vi "Periodic Tasks.vi"(8 "error in":errorcluster, 11 "pt cluster":T3={"linear acuator left"={"DeviceStatus"={"status"=FALSE, "code"=0, "source"=""}, "Type"=enum."CAN", "PWM"={"PWM Channel"=enum."Invalid", "DeadBand"={"Name"="", "maxPositivePwm"=0, "minPositivePwm"=0, "centerPwm"=0, "maxNegativePwm"=0, "minNegativePwm"=0, "angularRange"=0}}, "CAN"={"Device Number"=5, "SetOutput VI Ref"=variant(refnum<vi> refnum), "GetOutput VI Ref"=variant(refnum<vi> refnum), "Enable VI Ref"=variant(refnum<vi> refnum), "Disable VI Ref"=variant(refnum<vi> refnum), "Data"=variant(cluster{"Ext ID":u32, "Status 0 Session Handle":u32, "Status 1 Session Handle":u32, "Param Session Handle":u32, "Param Cache ref":refnum<data-value>, "CAN Timeout":u32, "Status 2 Session Handle":u32, "Status 3 Session Handle":u32, "Inverted No WPILib":bool, "Has Configured Limit Sw":bool, "Has Configured Alt Encoder":bool, "Status 4 Session Handle":u32} {"Ext ID"=33882117, "Status 0 Session Handle"=33657, "Status 1 Session Handle"=33658, "Param Session Handle"=33661, "Param Cache ref"=refnum, "CAN Timeout"=10, "Status 2 Session Handle"=33659, "Status 3 Session Handle"=33660, "Inverted No WPILib"=FALSE, "Has Configured Limit Sw"=FALSE, "Has Configured Alt Encoder"=FALSE, "Status 4 Session Handle"=0})}, "Invert"=FALSE, "DIO PWM"={"PWM \"Enable\" Channel"=enum."Invalid", "DIOChannel"=enum."Invalid", "PWM Rate"=0.0}}, "arm extension"={"DeviceStatus"={"status"=FALSE, "code"=0, "source"=""}, "Type"=enum."CAN", "PWM"={"PWM Channel"=enum."Invalid", "DeadBand"={"Name"="", "maxPositivePwm"=0, "minPositivePwm"=0, "centerPwm"=0, "maxNegativePwm"=0, "minNegativePwm"=0, "angularRange"=0}}, "CAN"={"Device Number"=7, "SetOutput VI Ref"=variant(refnum<vi> refnum), "GetOutput VI Ref"=variant(refnum<vi> refnum), "Enable VI Ref"=variant(refnum<vi> refnum), "Disable VI Ref"=variant(refnum<vi> refnum), "Data"=variant(cluster{"Ext ID":u32, "Status 0 Session Handle":u32, "Status 1 Session Handle":u32, "Param Session Handle":u32, "Param Cache ref":refnum<data-value>, "CAN Timeout":u32, "Status 2 Session Handle":u32, "Status 3 Session Handle":u32, "Inverted No WPILib":bool, "Has Configured Limit Sw":bool, "Has Configured Alt Encoder":bool, "Status 4 Session Handle":u32} {"Ext ID"=33882119, "Status 0 Session Handle"=33677, "Status 1 Session Handle"=33678, "Param Session Handle"=33681, "Param Cache ref"=refnum, "CAN Timeout"=10, "Status 2 Session Handle"=33679, "Status 3 Session Handle"=33680, "Inverted No WPILib"=FALSE, "Has Configured Limit Sw"=FALSE, "Has Configured Alt Encoder"=FALSE, "Status 4 Session Handle"=0})}, "Invert"=FALSE, "DIO PWM"={"PWM \"Enable\" Channel"=enum."Invalid", "DIOChannel"=enum."Invalid", "PWM Rate"=0.0}}, "turret"={"DeviceStatus"={"status"=FALSE, "code"=0, "source"=""}, "Type"=enum."CAN", "PWM"={"PWM Channel"=enum."Invalid", "DeadBand"={"Name"="", "maxPositivePwm"=0, "minPositivePwm"=0, "centerPwm"=0, "maxNegativePwm"=0, "minNegativePwm"=0, "angularRange"=0}}, "CAN"={"Device Number"=9, "SetOutput VI Ref"=variant(refnum<vi> refnum), "GetOutput VI Ref"=variant(refnum<vi> refnum), "Enable VI Ref"=variant(refnum<vi> refnum), "Disable VI Ref"=variant(refnum<vi> refnum), "Data"=variant(cluster{"Ext ID":u32, "Status 0 Session Handle":u32, "Status 1 Session Handle":u32, "Param Session Handle":u32, "Param Cache ref":refnum<data-value>, "CAN Timeout":u32, "Status 2 Session Handle":u32, "Status 3 Session Handle":u32, "Inverted No WPILib":bool, "Has Configured Limit Sw":bool, "Has Configured Alt Encoder":bool, "Status 4 Session Handle":u32} {"Ext ID"=33882121, "Status 0 Session Handle"=33651, "Status 1 Session Handle"=33652, "Param Session Handle"=33655, "Param Cache ref"=refnum, "CAN Timeout"=10, "Status 2 Session Handle"=33653, "Status 3 Session Handle"=33654, "Inverted No WPILib"=FALSE, "Has Configured Limit Sw"=FALSE, "Has Configured Alt Encoder"=FALSE, "Status 4 Session Handle"=0})}, "Invert"=FALSE, "DIO PWM"={"PWM \"Enable\" Channel"=enum."Invalid", "DIOChannel"=enum."Invalid", "PWM Rate"=0.0}}, "hood"={"DeviceStatus"={"status"=FALSE, "code"=0, "source"=""}, "Type"=enum."CAN", "PWM"={"PWM Channel"=enum."Invalid", "DeadBand"={"Name"="", "maxPositivePwm"=0, "minPositivePwm"=0, "centerPwm"=0, "maxNegativePwm"=0, "minNegativePwm"=0, "angularRange"=0}}, "CAN"={"Device Number"=14, "SetOutput VI Ref"=variant(refnum<vi> refnum), "GetOutput VI Ref"=variant(refnum<vi> refnum), "Enable VI Ref"=variant(refnum<vi> refnum), "Disable VI Ref"=variant(refnum<vi> refnum), "Data"=variant(cluster{"Ext ID":u32, "Status 0 Session Handle":u32, "Status 1 Session Handle":u32, "Param Session Handle":u32, "Param Cache ref":refnum<data-value>, "CAN Timeout":u32, "Status 2 Session Handle":u32, "Status 3 Session Handle":u32, "Inverted No WPILib":bool, "Has Configured Limit Sw":bool, "Has Configured Alt Encoder":bool, "Status 4 Session Handle":u32} {"Ext ID"=33882126, "Status 0 Session Handle"=33672, "Status 1 Session Handle"=33673, "Param Session Handle"=33676, "Param Cache ref"=refnum, "CAN Timeout"=10, "Status 2 Session Handle"=33674, "Status 3 Session Handle"=33675, "Inverted No WPILib"=FALSE, "Has Configured Limit Sw"=FALSE, "Has Configured Alt Encoder"=FALSE, "Status 4 Session Handle"=0})}, "Invert"=FALSE, "DIO PWM"={"PWM \"Enable\" Channel"=enum."Invalid", "DIOChannel"=enum."Invalid", "PWM Rate"=0.0}}, "climb brake"={"DevStatus"={"status"=FALSE, "code"=0, "source"=""}, "Pneumatics Control Module"=0, "Forward Solenoid Channel"=enum."Solenoid 4", "Reverse Solenoid Channel"=enum."Solenoid 5"}, "buddy climb"={"DevStatus"={"status"=FALSE, "code"=0, "source"=""}, "Pneumatics Control Module"=0, "Forward Solenoid Channel"=enum."Solenoid 6", "Reverse Solenoid Channel"=enum."Solenoid 7"}, "drivetrain shifter"={"DevStatus"={"status"=FALSE, "code"=0, "source"=""}, "Pneumatics Control Module"=0, "Forward Solenoid Channel"=enum."Solenoid 0", "Reverse Solenoid Channel"=enum."Solenoid 1"}, "hood"={"DevStatus"={"status"=FALSE, "code"=0, "source"=""}, "Pneumatics Control Module"=0, "Forward Solenoid Channel"=enum."Solenoid 1", "Reverse Solenoid Channel"=enum."Invalid"}, "climber encoder"={"DevStatus"={"status"=FALSE, "code"=0, "source"=""}, "EncoderIndex"=enum."Enc 2", "CounterIndex"=enum."Invalid", "DistancePerCount"=1.0, "Decoding Type"=enum."4x"}, "shooter encoder"={"DevStatus"={"status"=FALSE, "code"=0, "source"=""}, "EncoderIndex"=enum."Enc 3", "CounterIndex"=enum."Invalid", "DistancePerCount"=1.0, "Decoding Type"=enum."4x"}, "color sensor"={"I2CDevRef"={"DevStatus"={"status"=FALSE, "code"=0, "source"=""}, "Device Address"=82, "Handle"=54, "I2C Bus"=enum."I2C On-Board"}}, "linear acuator left pot"={"DevStatus"={"status"=FALSE, "code"=0, "source"=""}, "Analog Channel"=enum."AI 0", "Invert Output"=FALSE}, "linear acuator right pot "={"DevStatus"={"status"=FALSE, "code"=0, "source"=""}, "Analog Channel"=enum."AI 1", "Invert Output"=FALSE}, "auto balancer pot"={"DevStatus"={"status"=FALSE, "code"=0, "source"=""}, "Analog Channel"=enum."AI 3", "Invert Output"=FALSE}, "shooter"={"DeviceStatus"={"status"=FALSE, "code"=0, "source"=""}, "Type"=enum."CAN", "PWM"={"PWM Channel"=enum."Invalid", "DeadBand"={"Name"="", "maxPositivePwm"=0, "minPositivePwm"=0, "centerPwm"=0, "maxNegativePwm"=0, "minNegativePwm"=0, "angularRange"=0}}, "CAN"={"Device Number"=10, "SetOutput VI Ref"=variant(refnum<vi> refnum), "GetOutput VI Ref"=variant(refnum<vi> refnum), "Enable VI Ref"=variant(refnum<vi> refnum), "Disable VI Ref"=variant(refnum<vi> refnum), "Data"=variant(cluster{"Ext ID":u32, "Status 0 Session Handle":u32, "Status 1 Session Handle":u32, "Param Session Handle":u32, "Param Cache ref":refnum<data-value>, "CAN Timeout":u32, "Status 2 Session Handle":u32, "Status 3 Session Handle":u32, "Inverted No WPILib":bool, "Has Configured Limit Sw":bool, "Has Configured Alt Encoder":bool, "Status 4 Session Handle":u32} {"Ext ID"=33882122, "Status 0 Session Handle"=33689, "Status 1 Session Handle"=33690, "Param Session Handle"=33693, "Param Cache ref"=refnum, "CAN Timeout"=10, "Status 2 Session Handle"=33691, "Status 3 Session Handle"=33692, "Inverted No WPILib"=FALSE, "Has Configured Limit Sw"=FALSE, "Has Configured Alt Encoder"=FALSE, "Status 4 Session Handle"=0})}, "Invert"=FALSE, "DIO PWM"={"PWM \"Enable\" Channel"=enum."Invalid", "DIOChannel"=enum."Invalid", "PWM Rate"=0.0}}, "hopper"={"DeviceStatus"={"status"=FALSE, "code"=0, "source"=""}, "Type"=enum."CAN", "PWM"={"PWM Channel"=enum."PWM 1", "DeadBand"={"Name"="", "maxPositivePwm"=0, "minPositivePwm"=0, "centerPwm"=0, "maxNegativePwm"=0, "minNegativePwm"=0, "angularRange"=0}}, "CAN"={"Device Number"=12, "SetOutput VI Ref"=variant(refnum<vi> refnum), "GetOutput VI Ref"=variant(refnum<vi> refnum), "Enable VI Ref"=variant(refnum<vi> refnum), "Disable VI Ref"=variant(refnum<vi> refnum), "Data"=variant(cluster{"Library":path, "handle":u64, "Control Mode":u16, "UsageFrame":u32, "RefNumName":string, "arbID":u32} {"Library"=path "libCTRE_PhoenixCCI.so", "handle"=2979961472, "Control Mode"=0, "UsageFrame"=0, "RefNumName"="hopper", "arbID"=33816588})}, "Invert"=FALSE, "DIO PWM"={"PWM \"Enable\" Channel"=enum."Invalid", "DIOChannel"=enum."Invalid", "PWM Rate"=0.0}}, "feeder"={"DeviceStatus"={"status"=FALSE, "code"=0, "source"=""}, "Type"=enum."CAN", "PWM"={"PWM Channel"=enum."PWM 1", "DeadBand"={"Name"="", "maxPositivePwm"=0, "minPositivePwm"=0, "centerPwm"=0, "maxNegativePwm"=0, "minNegativePwm"=0, "angularRange"=0}}, "CAN"={"Device Number"=13, "SetOutput VI Ref"=variant(refnum<vi> refnum), "GetOutput VI Ref"=variant(refnum<vi> refnum), "Enable VI Ref"=variant(refnum<vi> refnum), "Disable VI Ref"=variant(refnum<vi> refnum), "Data"=variant(cluster{"Library":path, "handle":u64, "Control Mode":u16, "UsageFrame":u32, "RefNumName":string, "arbID":u32} {"Library"=path "libCTRE_PhoenixCCI.so", "handle"=3034680992, "Control Mode"=0, "UsageFrame"=0, "RefNumName"="feeder", "arbID"=33816589})}, "Invert"=FALSE, "DIO PWM"={"PWM \"Enable\" Channel"=enum."Invalid", "DIOChannel"=enum."Invalid", "PWM Rate"=0.0}}, "intake"={"DeviceStatus"={"status"=FALSE, "code"=0, "source"=""}, "Type"=enum."CAN", "PWM"={"PWM Channel"=enum."PWM 1", "DeadBand"={"Name"="", "maxPositivePwm"=0, "minPositivePwm"=0, "centerPwm"=0, "maxNegativePwm"=0, "minNegativePwm"=0, "angularRange"=0}}, "CAN"={"Device Number"=15, "SetOutput VI Ref"=variant(refnum<vi> refnum), "GetOutput VI Ref"=variant(refnum<vi> refnum), "Enable VI Ref"=variant(refnum<vi> refnum), "Disable VI Ref"=variant(refnum<vi> refnum), "Data"=variant(cluster{"Library":path, "handle":u64, "Control Mode":u16, "UsageFrame":u32, "RefNumName":string, "arbID":u32} {"Library"=path "libCTRE_PhoenixCCI.so", "handle"=42728016, "Control Mode"=0, "UsageFrame"=0, "RefNumName"="intake", "arbID"=33816591})}, "Invert"=FALSE, "DIO PWM"={"PWM \"Enable\" Channel"=enum."Invalid", "DIOChannel"=enum."Invalid", "PWM Rate"=0.0}}, "auto balance"={"DeviceStatus"={"status"=FALSE, "code"=0, "source"=""}, "Type"=enum."PWM", "PWM"={"PWM Channel"=enum."Invalid", "DeadBand"={"Name"="", "maxPositivePwm"=0, "minPositivePwm"=0, "centerPwm"=0, "maxNegativePwm"=0, "minNegativePwm"=0, "angularRange"=0}}, "CAN"={"Device Number"=0, "SetOutput VI Ref"=variant(refnum<vi> refnum), "GetOutput VI Ref"=variant(refnum<vi> refnum), "Enable VI Ref"=variant(refnum<vi> refnum), "Disable VI Ref"=variant(refnum<vi> refnum), "Data"=variant}, "Invert"=FALSE, "DIO PWM"={"PWM \"Enable\" Channel"=enum."Invalid", "DIOChannel"=enum."Invalid", "PWM Rate"=0.0}}, "linear acuator right"={"DeviceStatus"={"status"=FALSE, "code"=0, "source"=""}, "Type"=enum."CAN", "PWM"={"PWM Channel"=enum."Invalid", "DeadBand"={"Name"="", "maxPositivePwm"=0, "minPositivePwm"=0, "centerPwm"=0, "maxNegativePwm"=0, "minNegativePwm"=0, "angularRange"=0}}, "CAN"={"Device Number"=6, "SetOutput VI Ref"=variant(refnum<vi> refnum), "GetOutput VI Ref"=variant(refnum<vi> refnum), "Enable VI Ref"=variant(refnum<vi> refnum), "Disable VI Ref"=variant(refnum<vi> refnum), "Data"=variant(cluster{"Ext ID":u32, "Status 0 Session Handle":u32, "Status 1 Session Handle":u32, "Param Session Handle":u32, "Param Cache ref":refnum<data-value>, "CAN Timeout":u32, "Status 2 Session Handle":u32, "Status 3 Session Handle":u32, "Inverted No WPILib":bool, "Has Configured Limit Sw":bool, "Has Configured Alt Encoder":bool, "Status 4 Session Handle":u32} {"Ext ID"=33882118, "Status 0 Session Handle"=33662, "Status 1 Session Handle"=33663, "Param Session Handle"=33666, "Param Cache ref"=refnum, "CAN Timeout"=10, "Status 2 Session Handle"=33664, "Status 3 Session Handle"=33665, "Inverted No WPILib"=FALSE, "Has Configured Limit Sw"=FALSE, "Has Configured Alt Encoder"=FALSE, "Status 4 Session Handle"=0})}, "Invert"=FALSE, "DIO PWM"={"PWM \"Enable\" Channel"=enum."Invalid", "DIOChannel"=enum."Invalid", "PWM Rate"=0.0}}} {"color sensor"."I2CDevRef"."Device Address" format="%.0x"}) -> ()   [LabVIEW 2019]
doc: "This VI runs in parallel to other tasks. It can contain as many user-defined periodic loops as you need. These can carry out PID or other sorts of timed response."
uses:
  ptclustergood.ctl
  <vilib>/Rock Robotics/WPI/MotorControl/WPI_MotorControlDeviceRef.ctl
  <vilib>/Rock Robotics/WPI/MotorControl/WPI_MotorControlType.ctl
  <vilib>/Rock Robotics/SystemInterfaces/DIO/FPGA_DIOPWMChannel.ctl
  <vilib>/Rock Robotics/WPI/PWM/WPI_PWMDeadband.ctl
  <vilib>/Rock Robotics/SystemInterfaces/DIO/FPGA_DIOChannel.ctl
  <vilib>/Rock Robotics/WPI/Solenoid/WPI_SolenoidDevRef.ctl
  <vilib>/Rock Robotics/WPI/Solenoid/WPI_SolenoidChannel.ctl
  <vilib>/Rock Robotics/WPI/Encoder/WPI_EncoderDevRef.ctl
  <vilib>/Rock Robotics/SystemInterfaces/Encoder/FPGA_EncoderIdx.ctl
  <vilib>/Rock Robotics/SystemInterfaces/Counter/FPGA_CounterCtrSystemIndex.ctl
  <vilib>/Rock Robotics/WPI/Encoder/WPI_EncoderType.ctl
  <vilib>/Rock Robotics/WPI/ThirdParty/REV Robotics/Color SensorV3/Typedef/Color Sensor V3 DevRef.ctl
  <vilib>/Rock Robotics/WPI/I2C/WPI_I2CDevRef.ctl
  <vilib>/Rock Robotics/SystemInterfaces/i2clib/i2c_bus.ctl
  <vilib>/Rock Robotics/WPI/Potentiometer/WPI_PotentiometerDevRef.ctl
  <vilib>/Rock Robotics/SystemInterfaces/AI/FPGA_AIChannel.ctl
  <vilib>/Rock Robotics/WPI/ThirdParty/REV Robotics/SPARK MAX/Typedef/Spark MAX Control Type.ctl
  GlobalVariables.vi
  <vilib>/Rock Robotics/Network Tables/NT Read Number.vi
  <vilib>/addons/control/pid/pid.llb/PID (DBL).vi
  <vilib>/Rock Robotics/Network Tables/NT Write Number.vi
  <vilib>/addons/control/pid/NI_PID_pid.lvlib
panel:
  out "Shooter in range?":bool
  out "Crash Avoidance":bool
  in  "PID Constants hood":T1={"P Gain"=0.0, "I Gain"=0.0, "D Gain"=0.0, "F Gain"=0.0, "I Zone"=0.0, "Min Output"=-1.0, "Max Output"=1.0} {"Max Output" min=-1.0 max=1.0 step=0.01; "Min Output" min=-1.0 max=1.0 step=0.01; "I Zone" step=0.01; "F Gain" step=0.01; "D Gain" step=0.01; "I Gain" step=0.01; "P Gain" min=0.0 step=0.01}
  in  "offset zone 1":dbl
  in  "offset zone 3":dbl
  in  "setpoint":dbl=4800.0 format="%#_13g"
  in  "shooting":dbl=3.0
  in  "control panel lin act offset":dbl=0.25
  in  "min RPM":dbl=4100.0
  out "Sensor Velocity":dbl
  in  "No Color":cluster{"R":dbl, "G":dbl, "B":dbl}={"R"=80.0, "G"=119.0, "B"=55.0}
  in  "Yellow":cluster{"R":dbl, "G":dbl, "B":dbl}={"R"=83.0, "G"=130.0, "B"=41.0}
  in  "Blue":cluster{"R":dbl, "G":dbl, "B":dbl}={"R"=51.0, "G"=115.0, "B"=88.0}
  in  "Red":cluster{"R":dbl, "G":dbl, "B":dbl}={"R"=103.0, "G"=104.0, "B"=49.0}
  in  "Green":cluster{"R":dbl, "G":dbl, "B":dbl}={"R"=59.0, "G"=132.0, "B"=64.0}
  out "Confidence":dbl=0.9468771343442995
  out "Matched Color Name":string="Red"
  out "Proximity":u16=88
  out "Measured Color":cluster{"R":dbl, "G":dbl, "B":dbl}={"R"=91.53846153846153, "G"=108.97435897435896, "B"=54.48717948717948}
  out "Color":u32(colorbox)=6057270
  in  "PID Constants shooter":T1={"P Gain"=0.00141, "I Gain"=0.0, "D Gain"=0.0, "F Gain"=0.0004, "I Zone"=0.0, "Min Output"=0.0, "Max Output"=1.0} {"Max Output" min=-1.0 max=1.0 step=0.01; "Min Output" min=-1.0 max=1.0 step=0.01; "I Zone" step=0.01; "F Gain" step=0.01; "D Gain" step=0.01; "I Gain" step=0.01; "P Gain" min=0.0 step=0.01}
  in  "protect":dbl=0.2
  in  "offset zone 2":dbl
  in  "trench":dbl=41.3
  in  "layup":dbl=1.0
  in  "Hood Gains":T2={"proportional gain (Kc)"=0.1, "integral time (Ti, min)"=0.0, "derivative time (Td, min)"=0.0} {"derivative time (Td, min)" format="%.3f"; "integral time (Ti, min)" format="%.3f"; "proportional gain (Kc)" format="%.5f"}
  in  "degrees per click hood":dbl=0.278416
  out "hood degrees":dbl=28.823331198364258
  in  "Shooter Gains":T2={"proportional gain (Kc)"=2.0, "integral time (Ti, min)"=0.0, "derivative time (Td, min)"=0.0} {"derivative time (Td, min)" format="%.3f"; "integral time (Ti, min)" format="%.3f"; "proportional gain (Kc)" format="%.3f"}
  in  "lower limit":dbl=-270.0 format="%#_13g"
  in  "upper limit":dbl format="%#_13g"
  in  "Minimum Track Value Turret":dbl=0.05 format="%#_13g"
  in  "Auto Correct Gain Turret":dbl=1.2 format="%#_13g"
  in  "X Accepted Range Turret":dbl
  in  "Backward":dbl
  in  "Forward":dbl=-180.0
  in  "Arm Extension Gains":T2={"proportional gain (Kc)"=0.15, "integral time (Ti, min)"=0.0, "derivative time (Td, min)"=0.0} {"derivative time (Td, min)" format="%.3f"; "integral time (Ti, min)" format="%.3f"; "proportional gain (Kc)" format="%.5f"}
  in  "Turret Gains":T2={"proportional gain (Kc)"=0.025, "integral time (Ti, min)"=0.0, "derivative time (Td, min)"=0.0} {"derivative time (Td, min)" format="%.3f"; "integral time (Ti, min)" format="%.3f"; "proportional gain (Kc)" format="%.5f"}
  in  "degrees per click turret":dbl=1.65
  out "RPM":dbl
  in  "Acuator Gains":T2={"proportional gain (Kc)"=0.3, "integral time (Ti, min)"=0.0, "derivative time (Td, min)"=0.0} {"derivative time (Td, min)" format="%.3f"; "integral time (Ti, min)" format="%.3f"; "proportional gain (Kc)" format="%.5f"}
  in  "right act value at 1 inch":dbl=0.919
  out "right act pos":dbl=-0.2551903082312883
  out "left act pos":dbl=-0.2307307128952676
  in  "left act value at 1 inch":dbl=0.919
  in  "Inches per volt":dbl=13.5
  out "acuator left":dbl=0.936091163918168
  out "acuator right":dbl=0.9379029857949104
  out "turret degrees":dbl=-0.43214263468980785
  in  "clicks per inch arm":dbl=0.251624
  in  "control panel":dbl=5.0
  in  "climb":dbl=10.5
  in  "Ground":dbl=-0.3
  out "Arm Extension Encoder":dbl=5.206198121124268
  in  "climb":dbl=19.0
  in  "control panel":dbl=8.0
  in  "intake":dbl=8.5
  in  "protect":dbl=2.0
  # "Arm Height"
  # "Arm Extension"
  # "Linear Acuator Controls"
  # "Practice Bot\nLeft : .88\nRight : .886\n\nComb Bot\nLeft : .919\nRight : .919"
  # "Shooter"
  # "Click here to set max"
  # "Click here to set min"
  # "Click here to set max"
  # "Click here to set min"
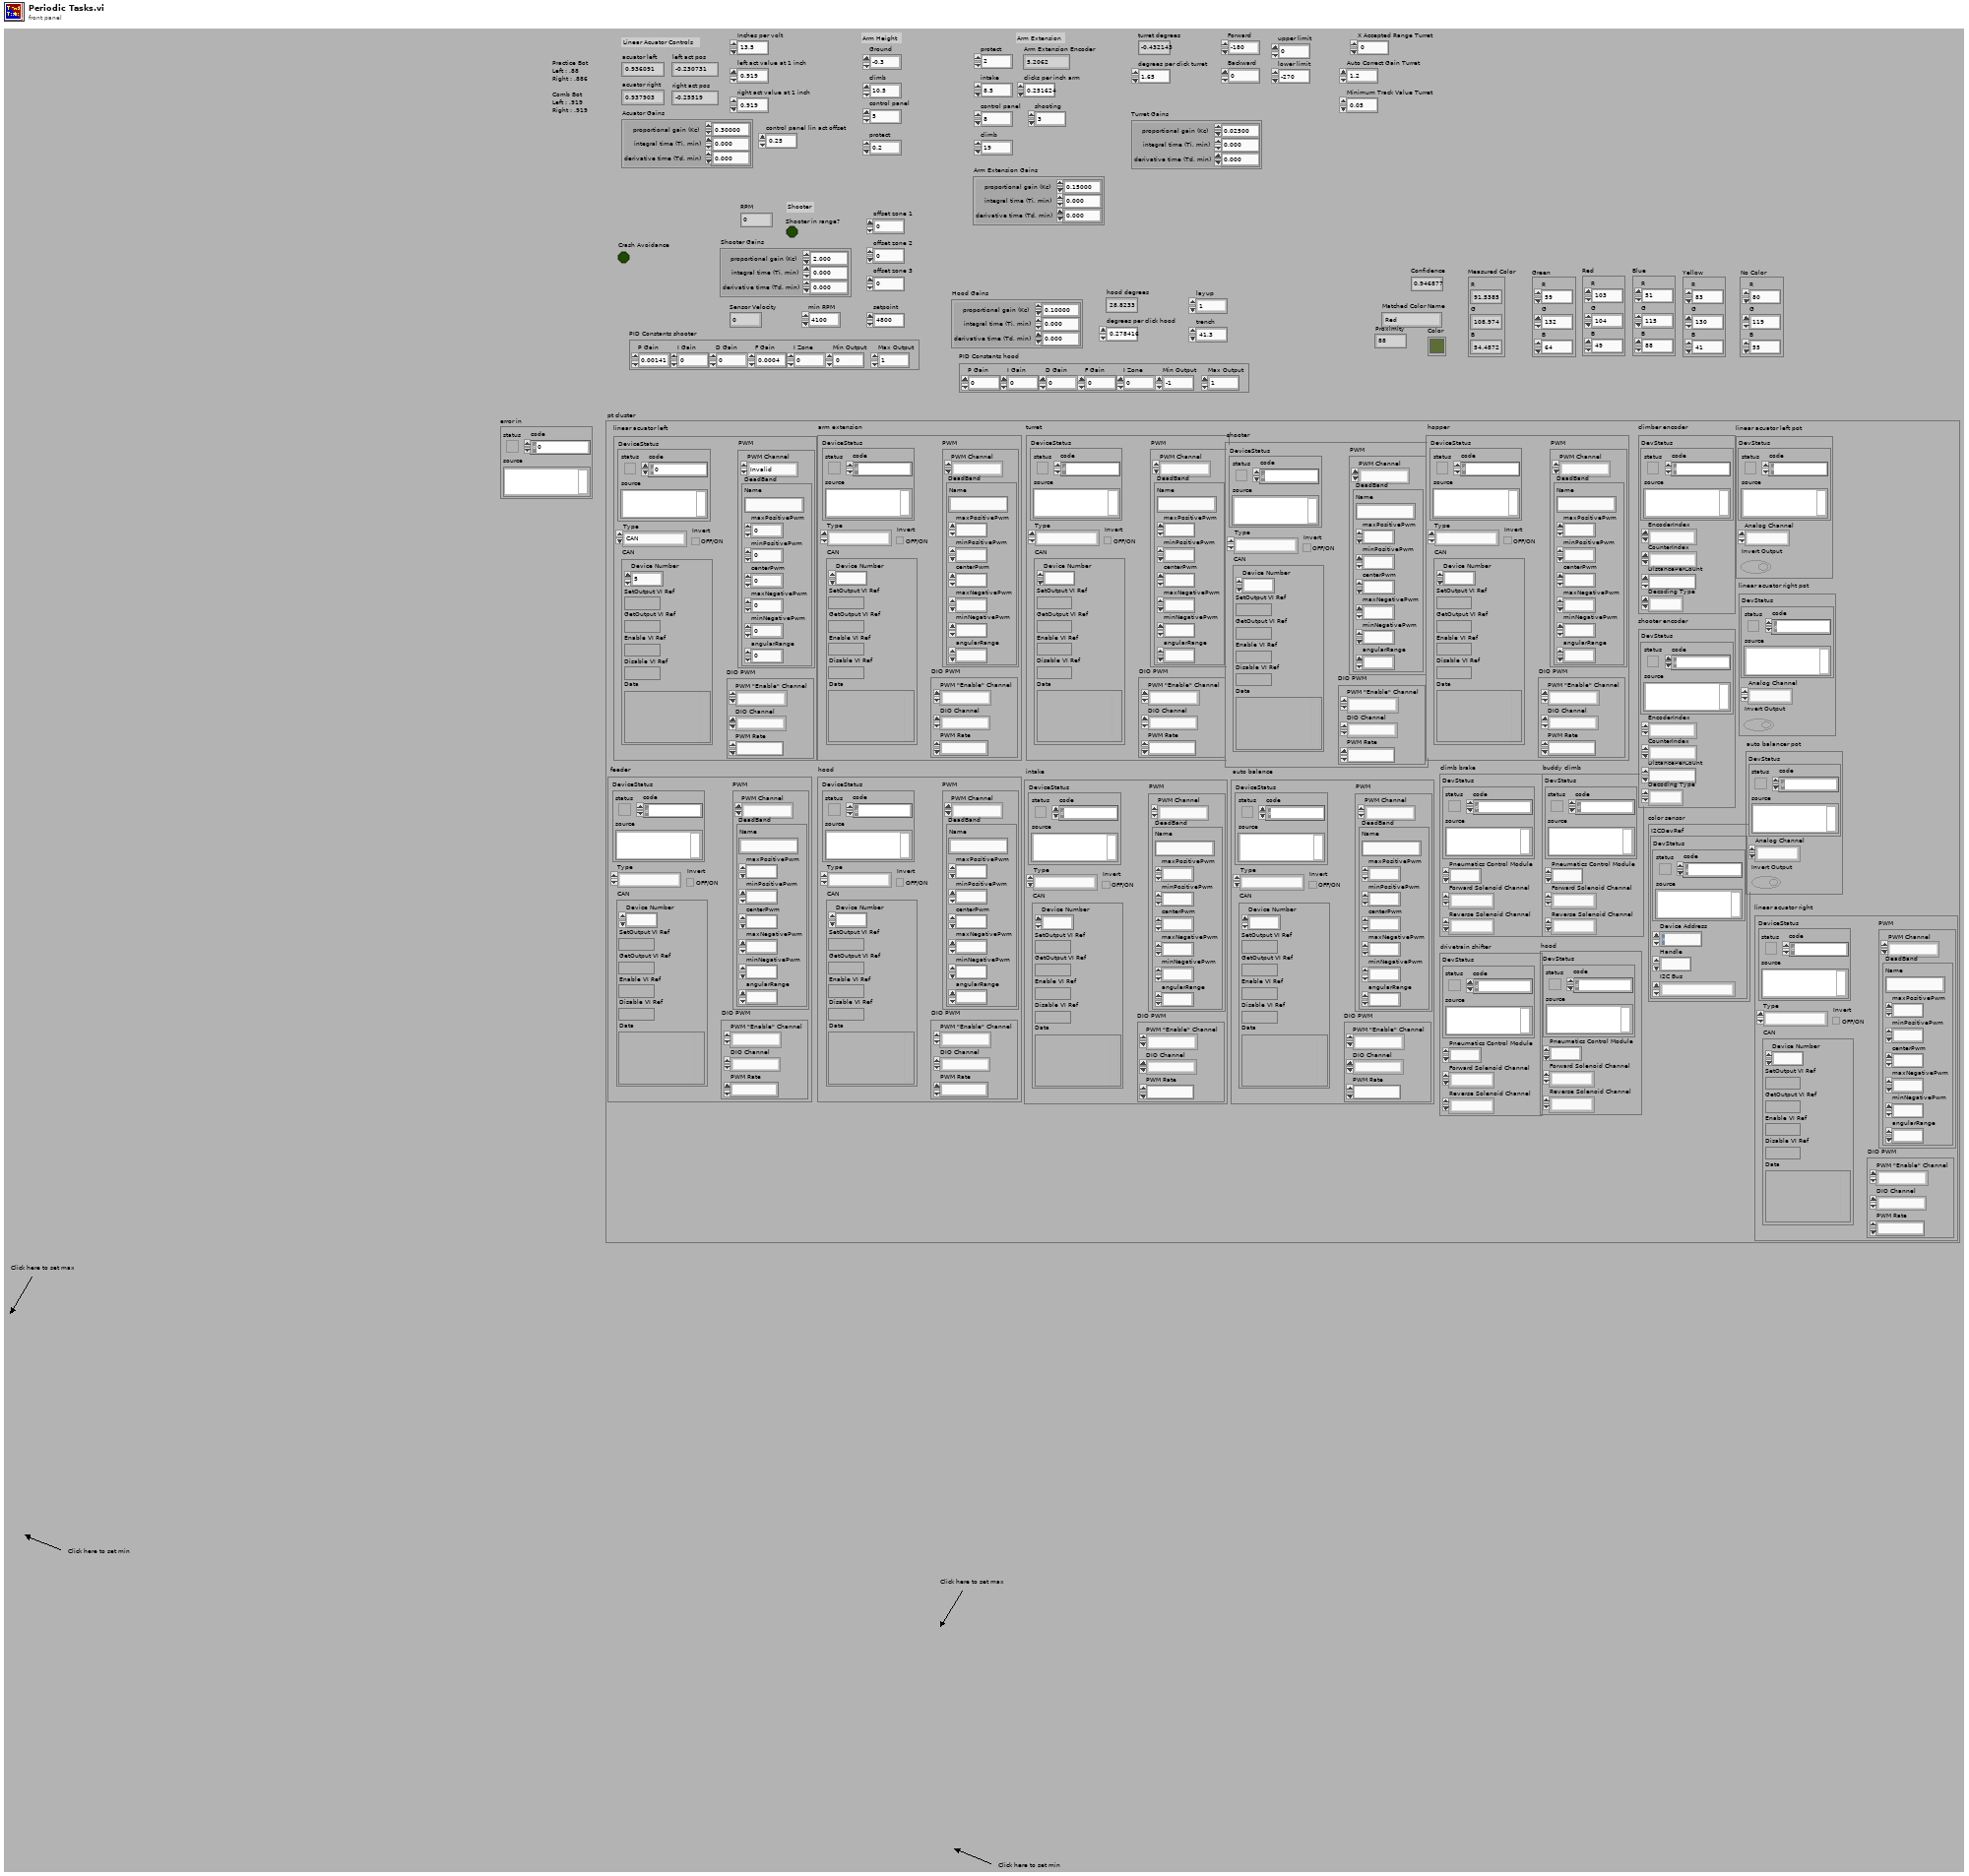
[diagram p1: front panel]
types:
  T1 = cluster{"P Gain":dbl, "I Gain":dbl, "D Gain":dbl, "F Gain":dbl, "I Zone":dbl, "Min Output":dbl, "Max Output":dbl}
  T2 = cluster{"proportional gain (Kc)":dbl, "integral time (Ti, min)":dbl, "derivative time (Td, min)":dbl}
  T3 = typedef "ptclustergood.ctl" = cluster{"linear acuator left":T4, "arm extension":T4, "turret":T4, "hood":T4, "climb brake":T9, "buddy climb":T9, "drivetrain shifter":T9, "hood":T9, "climber encoder":T11, "shooter encoder":T11, "color sensor":T15, "linear acuator left pot":T18, "linear acuator right pot ":T18, "auto balancer pot":T18, "shooter":T4, "hopper":T4, "feeder":T4, "intake":T4, "auto balance":T4, "linear acuator right":T4}
  T4 = typedef "WPI_MotorControlDeviceRef.ctl" = cluster{"DeviceStatus":errorcluster, "Type":T5, "PWM":cluster{"PWM Channel":T6, "DeadBand":T7}, "CAN":cluster{"Device Number":u8, "SetOutput VI Ref":variant, "GetOutput VI Ref":variant, "Enable VI Ref":variant, "Disable VI Ref":variant, "Data":variant}, "Invert":bool, "DIO PWM":cluster{"PWM \"Enable\" Channel":T6, "DIOChannel":T8, "PWM Rate":dbl}}
  T5 = typedef "WPI_MotorControlType.ctl" = enum16{"PWM", "CAN", "DIO PWM"}
  T6 = typedef "FPGA_DIOPWMChannel.ctl" = enum8{"PWM 0", "PWM 1", "PWM 2", "PWM 3", "PWM 4", "PWM 5", "PWM 6", "PWM 7", "PWM 8", "PWM 9", "PWM MXP 0", "PWM MXP 1", "PWM MXP 2", "PWM MXP 3", "PWM MXP 4", "PWM MXP 5", "PWM MXP 6", "PWM MXP 7", "PWM MXP 8", "PWM MXP 9", "Invalid"}
  T7 = typedef "WPI_PWMDeadband.ctl" = cluster{"Name":string, "maxPositivePwm":i32, "minPositivePwm":i32, "centerPwm":i32, "maxNegativePwm":i32, "minNegativePwm":i32, "angularRange":u16}
  T8 = typedef "FPGA_DIOChannel.ctl" = enum8{"DIO 0", "DIO 1", "DIO 2", "DIO 3", "DIO 4", "DIO 5", "DIO 6", "DIO 7", "DIO 8", "DIO 9", "DIO MXP 0", "DIO MXP 1", "DIO MXP 2", "DIO MXP 3", "DIO MXP 4", "DIO MXP 5", "DIO MXP 6", "DIO MXP 7", "DIO MXP 8", "DIO MXP 9", "DIO MXP 10", "DIO MXP 11", "DIO MXP 12", "DIO MXP 13", "DIO MXP 14", "DIO MXP 15", "SPI Port CS1", "SPI Port CS2", "SPI Port CS3", "SPI Port MISO", "SPI Port MOSI", "Invalid"}
  T9 = typedef "WPI_SolenoidDevRef.ctl" = cluster{"DevStatus":errorcluster, "Pneumatics Control Module":u8, "Forward Solenoid Channel":T10, "Reverse Solenoid Channel":T10}
  T10 = typedef "WPI_SolenoidChannel.ctl" = enum8{"Solenoid 0", "Solenoid 1", "Solenoid 2", "Solenoid 3", "Solenoid 4", "Solenoid 5", "Solenoid 6", "Solenoid 7", "Invalid"}
  T11 = typedef "WPI_EncoderDevRef.ctl" = cluster{"DevStatus":errorcluster, "EncoderIndex":T12, "CounterIndex":T13, "DistancePerCount":dbl, "Decoding Type":T14}
  T12 = typedef "FPGA_EncoderIdx.ctl" = enum8{"Enc 0", "Enc 1", "Enc 2", "Enc 3", "Enc 4", "Enc 5", "Enc 6", "Enc 7", "Invalid"}
  T13 = typedef "FPGA_CounterCtrSystemIndex.ctl" = enum8{"Ctr 0", "Ctr 1", "Ctr 2", "Ctr 3", "Ctr 4", "Ctr 5", "Ctr 6", "Ctr 7", "Invalid"}
  T14 = typedef "WPI_EncoderType.ctl" = enum16{"1x", "2x", "4x"}
  T15 = typedef "Color Sensor V3 DevRef.ctl" = cluster{"I2CDevRef":T16}
  T16 = typedef "WPI_I2CDevRef.ctl" = cluster{"DevStatus":errorcluster, "Device Address":u8, "Handle":i32, "I2C Bus":T17}
  T17 = typedef "i2c_bus.ctl" = enum16{"I2C On-Board", "I2C MXP", "Invalid"}
  T18 = typedef "WPI_PotentiometerDevRef.ctl" = cluster{"DevStatus":errorcluster, "Analog Channel":T19, "Invert Output":bool}
  T19 = typedef "FPGA_AIChannel.ctl" = enum8{"AI 0", "AI 1", "AI 2", "AI 3", "AI MXP 0", "AI MXP 1", "AI MXP 2", "AI MXP 3", "Invalid"}
  T20 = typedef "WPI_AnalogChannelDevRef.ctl" = cluster{"DevStatus":errorcluster, "Analog Channel":T19}
  T21 = typedef "Spark MAX Control Type.ctl" = enum16{"Percent VBus", "Voltage", "Velocity", "Position", "Smart Motion", "Current", "Smart Velocity"}
  T22 = enum16{"ground protect", "ground pickup", "control panel", "shooting", "climb", "unjam", "intake shoot"}
  T23 = enum16{"intake", "protect", "control", "climb", "shooting"}
  T24 = enum16{"ground", "protect", "climb", "control panel"}
  T25 = cluster{"P Gain":bool, "I Gain":bool, "D Gain":bool, "F Gain":bool, "I Zone":bool, "Min Output":bool, "Max Output":bool}
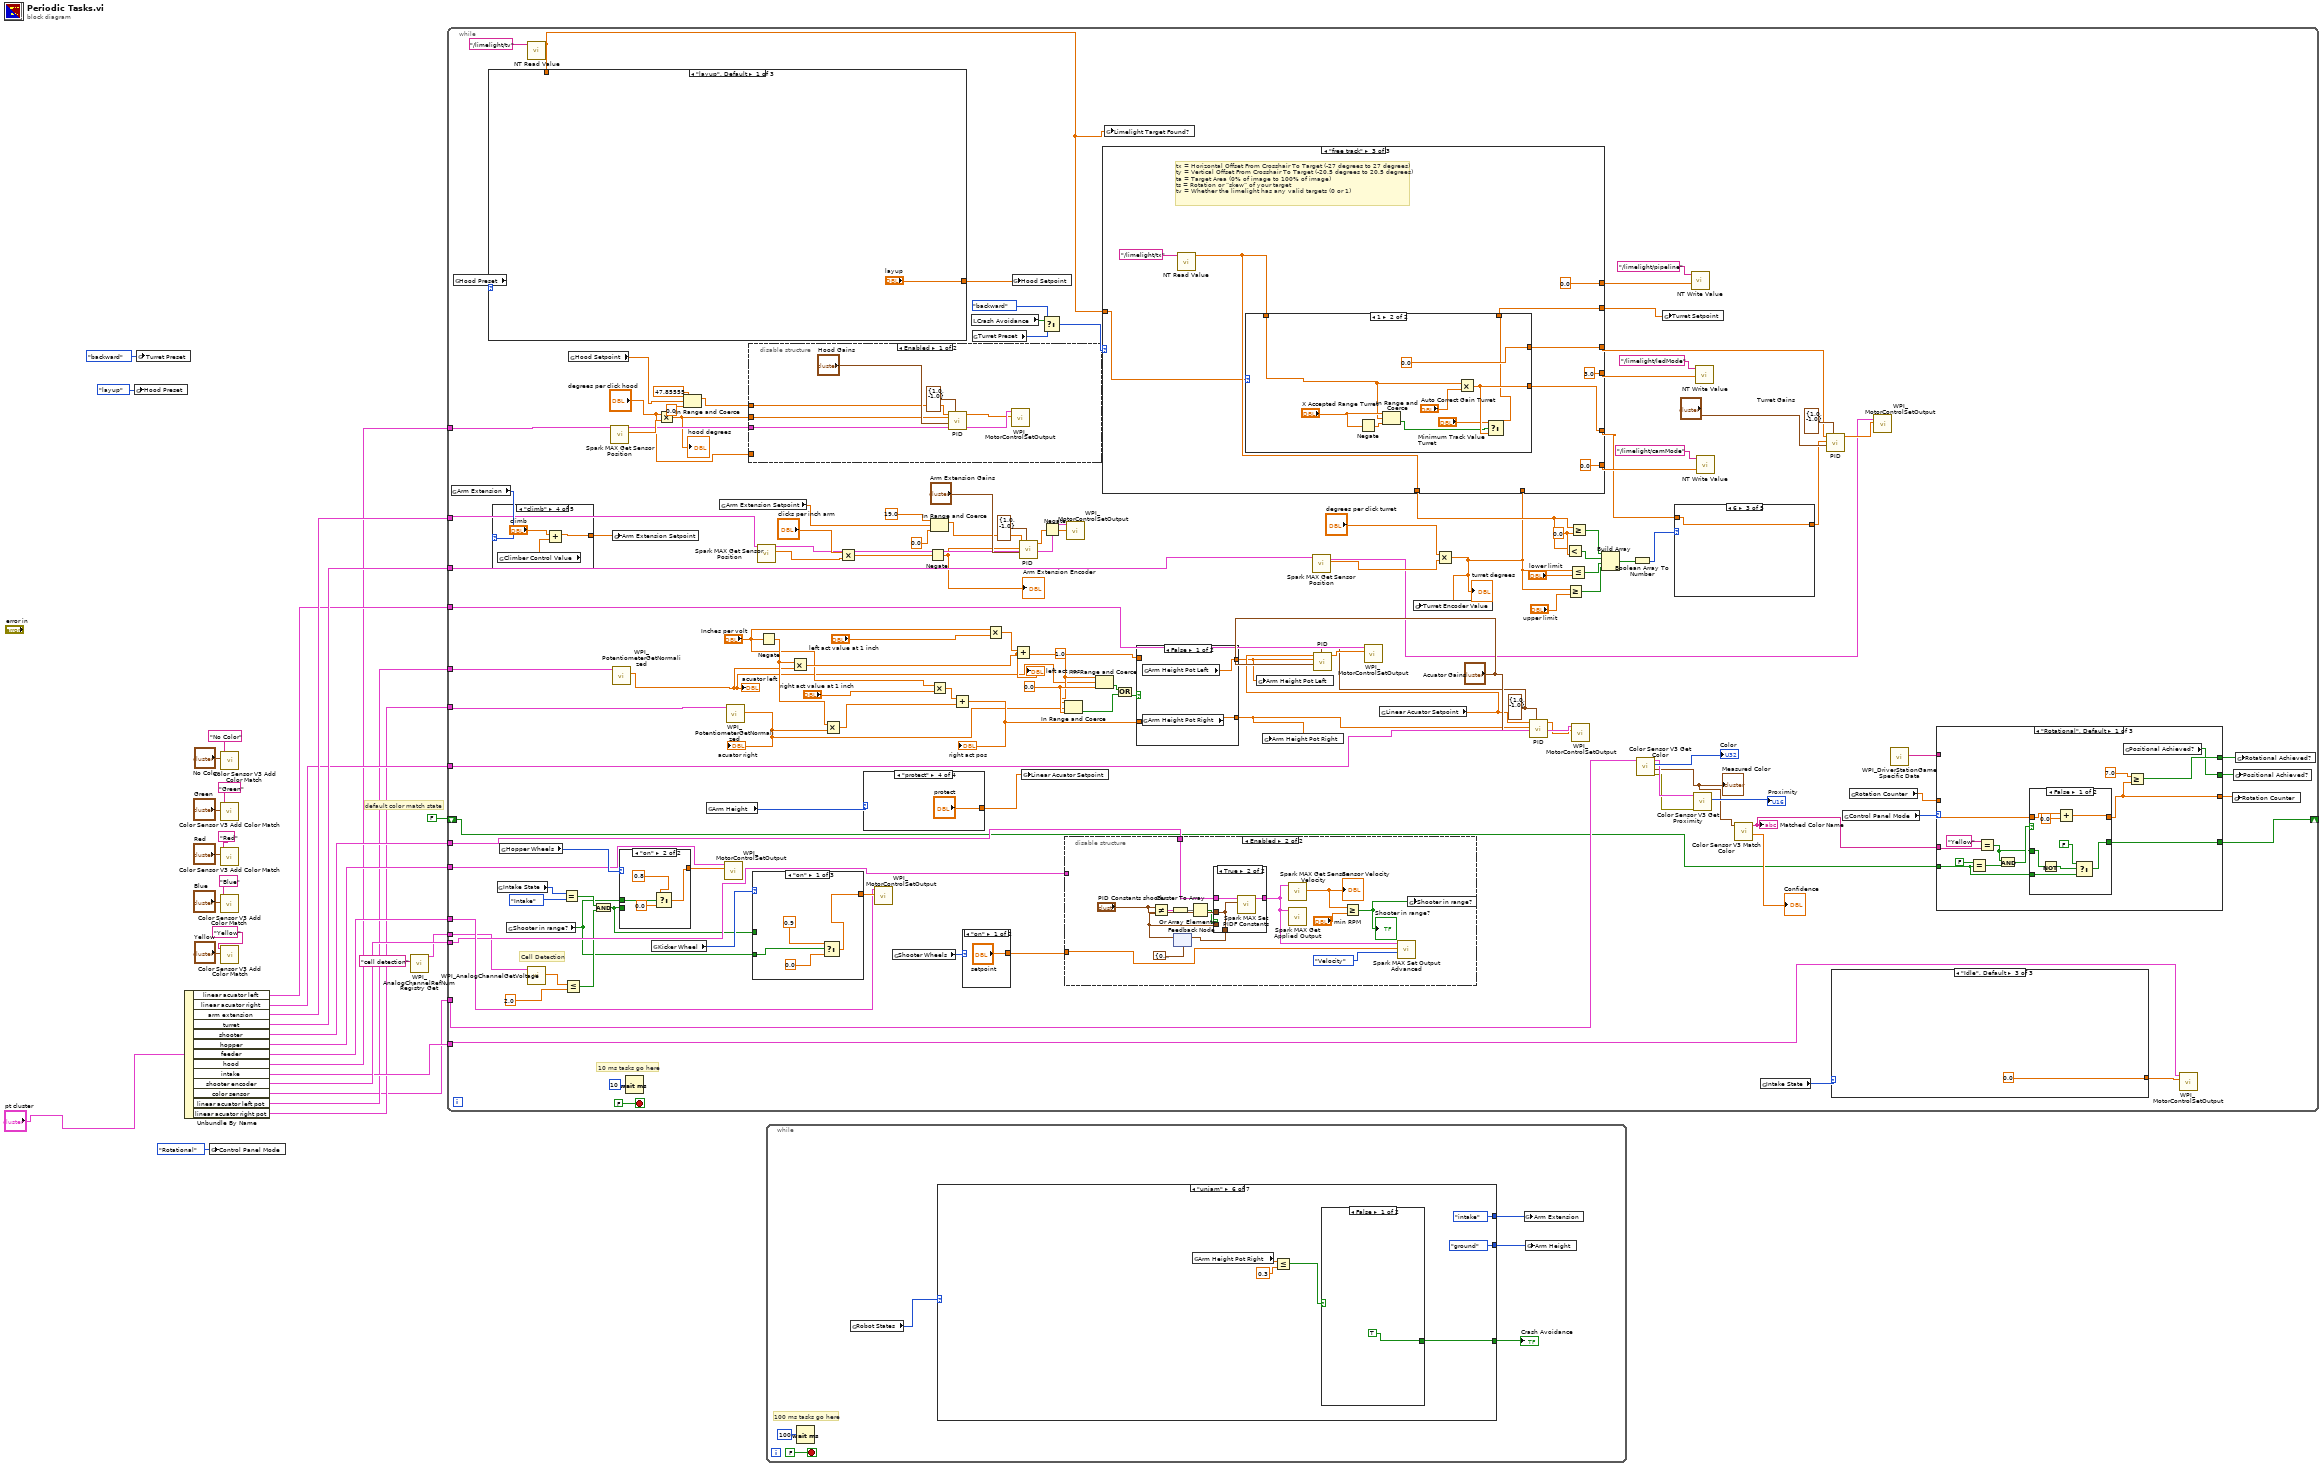
[diagram p0: block diagram]
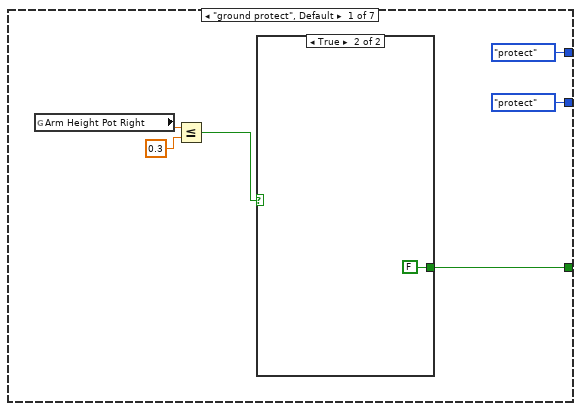
[diagram p2: hidden frame]
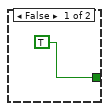
[diagram p3: hidden frame]
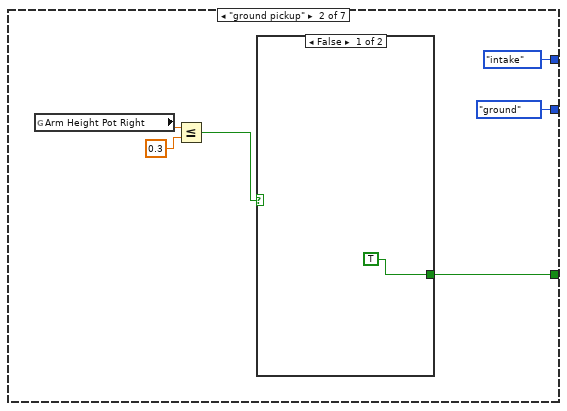
[diagram p4: hidden frame]
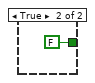
[diagram p5: hidden frame]
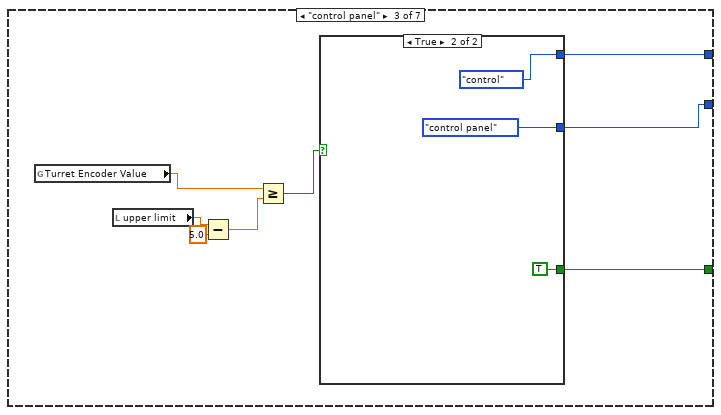
[diagram p6: hidden frame]
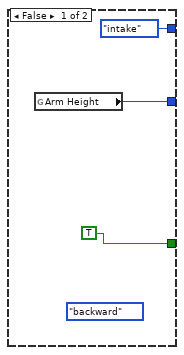
[diagram p7: hidden frame]
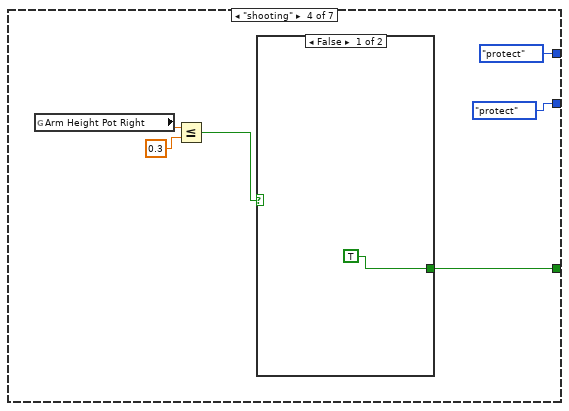
[diagram p8: hidden frame]
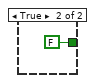
[diagram p9: hidden frame]
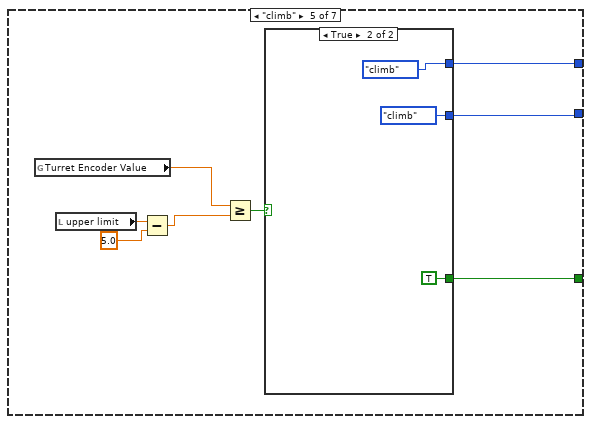
[diagram p10: hidden frame]
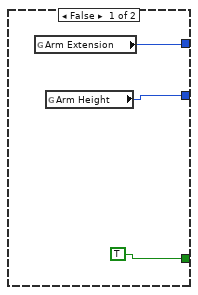
[diagram p11: hidden frame]
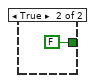
[diagram p12: hidden frame]
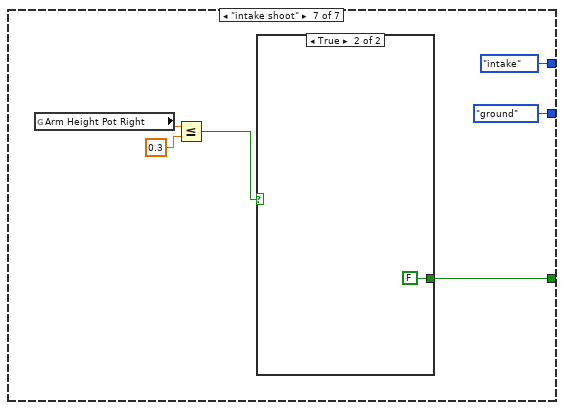
[diagram p13: hidden frame]
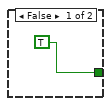
[diagram p14: hidden frame]
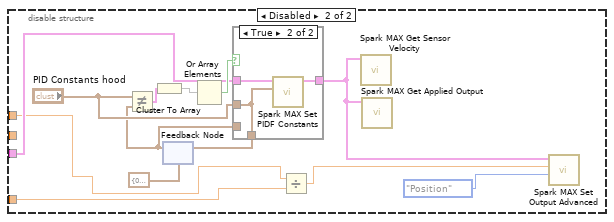
[diagram p15: hidden frame]
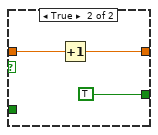
[diagram p18: hidden frame]
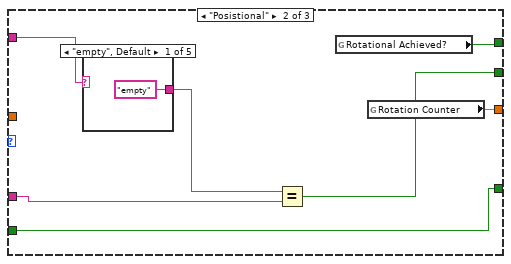
[diagram p19: hidden frame]
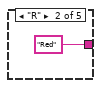
[diagram p20: hidden frame]
diagram:
  # "default color match state"
  n1 = global write "GlobalVariables.vi" "Hood Preset"(enum16{"trench", "layup", "free track"}."layup" ("Hood Preset")) -> ()
  n2 = global write "GlobalVariables.vi" "Turret Preset"(enum16{"free track", "forward", "backward"}."backward" ("Turret Preset")) -> ()
  n3 = Unbundle By Name("pt cluster") -> ("linear acuator left"=w21:T4, "linear acuator right"=w22:T4, "arm extension"=w28:T4, "turret"=w24:T4, "shooter"=w26:T4, "hopper"=w29:T4, "feeder"=w30:T4, "hood"=w17:T4, "intake"=w25:T4, "shooter encoder"=w27:T11, "color sensor"=w18:T15, "linear acuator left pot"=w20:T18, "linear acuator right pot"=w19:T18)
  n4 = global write "GlobalVariables.vi" "Control Panel Mode"(enum16{"Rotational", "None", "Posistional"}."Rotational" ("Control Panel Mode")) -> ()
  n5 = call <vilib>:"Color Sensor V3 Add Color Match.vi"("Color"="Green", "Name"="Green") -> ()  [unwired: 10 in]
  n6 = call <vilib>:"Color Sensor V3 Add Color Match.vi"("Color"="Red", "Name"="Red") -> ()  [unwired: 10 in]
  n7 = call <vilib>:"Color Sensor V3 Add Color Match.vi"("Color"="Blue", "Name"="Blue") -> ()  [unwired: 10 in]
  n8 = call <vilib>:"Color Sensor V3 Add Color Match.vi"("Color"="No Color", "Name"="No Color") -> ()  [unwired: 10 in]
  n9 = call <vilib>:"Color Sensor V3 Add Color Match.vi"("Color"="Yellow", "Name"="Yellow") -> ()  [unwired: 10 in]
  n10 = call <vilib>:"WPI_AnalogChannelRefNum Registry Get.vi"("refnum name"="cell detection") -> ("AIDeviceRef"=w3:T20)  [unwired: 9 in, 1 out]
  n11 = while {
    tunnel: w19 -> [w158]
    tunnel: w29 -> [w154]
    tunnel: w30 -> [w151]
    tunnel: w28 -> [w150]
    tunnel: w27 -> [w118]
    tunnel: w26 -> [w81]
    tunnel: w18 -> [w84]
    tunnel: w25 -> [w144]
    tunnel: w24 -> [w138]
    tunnel: w20 -> [w134]
    tunnel: w22 -> [w125]
    tunnel: w21 -> [w120]
    tunnel: w17 -> [w91]
    shift-right: [w70] -> _
    shift-left: FALSE -> [w71]
    tunnel: w3 -> [w55]
    stop <- FALSE stop-if-true
    w43 = 0.0 ("lower limit")
    w40 = 1.0 ("upper limit")
    w97 = 0.0 ("y")
    w119 = cluster{"output high":dbl, "output low":dbl} {"output high"=1.0, "output low"=-1.0} ("output range")
    # "Cell Detection"
    # "10 ms tasks go here"
    n12 = global read "GlobalVariables.vi" "Arm Extension"() -> (w159:T23)
    n13 = global read "GlobalVariables.vi" "Hood Preset"() -> (w89:enum16{"trench", "layup", "free track"})
    n14 = case shown="\"climb\"" w159 {
      tunnel: ["protect" "intake" "control panel" w385 "shooting"] -> w143
      frame "protect" {
      }
      frame "intake" {
      }
      frame "control" {
      }
      frame "climb" {
        n15 = global read "GlobalVariables.vi" "Climber Control Value"() -> (w384:dbl)
        n16 = Add(x="climb", y=w384) -> (x+y=w385:dbl)
      }
      frame "shooting" {
      }
    }
    n17 = global read "GlobalVariables.vi" "Intake State"() -> (w54:enum16{"Idle", "Intake", "Spit"})
    n18 = global read "GlobalVariables.vi" "Hopper Wheels"() -> (w155:enum16{"on", "off"})
    n19 = global read "GlobalVariables.vi" "Shooter in range?"() -> (w31:bool)
    n20 = call-poly <vilib>:"NT Read Value.vi"("Name"="/limelight/tv") -> ("Numeric"=w32:dbl)  [unwired: 9 in, 1 out]
    n21 = case shown="\"layup\", Default" w89 {
      tunnel: ["layup" "trench" w265] -> w88
      tunnel: w32 -> [_ _ w269]
      frame "layup", Default {
      }
      frame "trench" {
      }
      frame "free track" {
        n22 = call-poly <vilib>:"NT Read Value.vi"("Name"="/limelight/ty") -> ("Numeric"=w270:dbl)  [unwired: 9 in, 1 out]
        n23 = case shown="1" w269 {
          tunnel: [w273 w291] -> w267
          tunnel: w270 -> [_ w277]
          tunnel: [0.0 ("offset zone 3") w274] -> w266
          frame 0, Default {
            n24 = global read "GlobalVariables.vi" "Hood Setpoint"() -> (w273:dbl)
          }
          frame 1 {
            w278 = -12.0 ("y")
            w283 = -4.26 ("y")
            n25 = Less?(x=w277, y=w283) -> (x < y?=w285:bool)
            n26 = Greater Or Equal?(x=w277, y=w278) -> (x >= y?=w286:bool)
            n27 = Less?(x=w277, y=28.0 ("upper limit")) -> (x < y?=w289:bool)
            n28 = Greater Or Equal?(x=w277, y=w283) -> (x >= y?=w288:bool)
            n29 = Less?(x=w277, y=w278) -> (x < y?=w280:bool)
            n30 = Greater Or Equal?(x=w277, y=-28.0) -> (x >= y?=w281:bool)
            n31 = And(x=w285, y=w286) -> (x .and. y?=w284:bool)
            n32 = And(x=w289, y=w288) -> (x .and. y?=w287:bool)
            n33 = And(x=w280, y=w281) -> (x .and. y?=w279:bool)
            n34 = Build Array(w287, w284, w279) -> (w276:bool[])
            n35 = Boolean Array To Number(Boolean array=w276) -> (number=w275:u32)
            n36 = case shown="4" w275 {
              tunnel: [w294 w296 w299] -> w291
              tunnel: w277 -> [w293 w297 w300]
              tunnel: ["offset zone 1" "offset zone 2" "offset zone 3"] -> w274
              frame 1, Default {
                n37 = formula code="y = -0.405*x+30.872;"("x"=w293) -> ("y"=w294:dbl)
              }
              frame 2 {
                n38 = formula code="y = -0.405*x+30.872;"("x"=w297) -> ("y"=w296:dbl)
              }
              frame 4 {
                n39 = formula code="y = 0.0232*x*x*x*x + 1.2792*x*x*x + 25.945*x*x + 228.67*x + 773.62\n;"("x"=w300) -> ("y"=w299:dbl)
              }
            }
          }
        }
        n40 = Add(x=w267, y=w266) -> (x+y=w265:dbl)
        n41 = call "Slop Adjustment.vi"("Slop Measure"=5.0, "Adjustment"=w266) -> ()  [unwired: 9 in, 1 out]
      }
    }
    n42 = call <vilib>:"WPI_AnalogChannelGetVoltage.vi"("AIDeviceRef"=w55) -> ("Voltage"=w57:dbl)  [unwired: 8 in, 2 out]
    n43 = Equal?(x=w54, y=enum16{"Idle", "Intake", "Spit"}."Intake" ("Intake State")) -> (x = y?=w52:bool)
    n44 = Less Or Equal?(x=w57, y=2.0) -> (x <= y?=w51:bool)
    n45 = global read "GlobalVariables.vi" "Hood Setpoint"() -> (w64:dbl)
    n46 = And(x=w52, y=w51) -> (x .and. y?=w50:bool)
    n47 = call <vilib>:"Spark MAX Get Sensor Position.vi"("MotorControlDevRef in"=w91) -> ("Sensor Position"=w92:dbl, "MotorControlDevRef out"=w90:T4)  [unwired: 7 in, 2 out]
    n48 = global write "GlobalVariables.vi" "Arm Extension Setpoint"(w143) -> ()
    n49 = call <vilib>:"WPI_PotentiometerGetNormalized.vi"("PotDevRef"=w134) -> ("Normalized Value"=w39:dbl)  [unwired: 8 in, 2 out]
    "acuator left" <- w39
    n50 = case shown="\"on\"" w155 {
      tunnel: [w368 w373] -> w156
      tunnel: w50 -> [w371 _]
      tunnel: w31 -> [_ w375]
      frame "off", Default {
        n51 = Select(t=0.8 ("Output"), s=w371, f=0.0) -> (s? t:f=w368:dbl)
      }
      frame "on" {
        n52 = Select(t=0.8 ("Output"), s=w375, f=0.0) -> (s? t:f=w373:dbl)
      }
    }
    n53 = Wait (ms)(milliseconds to wait=u32 10) -> ()  [unwired: 1 out]
    n54 = global read "GlobalVariables.vi" "Kicker Wheel"() -> (w153:enum16{"on", "off", "reverse"})
    n55 = Multiply(x="degrees per click hood", y=w92) -> (x*y=w62:dbl)
    "hood degrees" <- w62
    n56 = In Range and Coerce(upper limit=47.85555, x=w64, lower limit=0.0) -> (coerced(x)=w63:dbl)  [unwired: 1 out]
    n57 = global read "GlobalVariables.vi" "Arm Height"() -> (w157:T24)
    n58 = global read "GlobalVariables.vi" "Arm Extension Setpoint"() -> (w61:dbl)
    n59 = call <vilib>:"WPI_MotorControlSetOutput.vi"("Output"=w156, "MotorControlDevRef"=w154) -> ()  [unwired: 7 in, 3 out]
    n60 = call <vilib>:"WPI_PotentiometerGetNormalized.vi"("PotDevRef"=w158) -> ("Normalized Value"=w38:dbl)  [unwired: 8 in, 2 out]
    "acuator right" <- w38
    n61 = disable-structure shown="Enabled" {
      disable-tunnel: w90 -> [w165 w171]
      disable-tunnel: w63 -> [w164 w170]
      disable-tunnel: w62 -> [w163 _]
      disable-tunnel: "degrees per click hood" -> [_ w168]
      frame Enabled {
        n62 = call-poly <vilib>:"PID.vi"("output range"=cluster{"output high":dbl, "output low":dbl} {"output high"=1.0, "output low"=-1.0}, "PID gains"="Hood Gains", "process variable"=w163, "setpoint"=w164) -> ("output"=w162:dbl)  [unwired: 6 in, 1 out]
        n63 = call <vilib>:"WPI_MotorControlSetOutput.vi"("Output"=w162, "MotorControlDevRef"=w165) -> ()  [unwired: 7 in, 3 out]
      }
      frame Disabled {
        n64 = feedback #1(T1 {"P Gain"=0.0, "I Gain"=0.0, "D Gain"=0.0, "F Gain"=0.0, "I Zone"=0.0, "Min Output"=0.0, "Max Output"=0.0} ("PID Constants")) -> (w175:T1)
        n65 = Not Equal?(x="PID Constants hood", y=w175) -> (x != y?=w179:T25)
        n66 = Cluster To Array(cluster=w179) -> (array=w178:bool[])
        n67 = Or Array Elements(Boolean array=w178) -> (logical OR=w177:bool)
        n68 = case shown="True" w177 {
          tunnel: "PID Constants hood" -> [_ w184]
          tunnel: [w182 w184] -> w172
          tunnel: w175 -> [w182 _]
          tunnel: [w181 w185] -> w180
          tunnel: w171 -> [w181 w183]
          frame False {
          }
          frame True {
            n69 = call <vilib>:"Spark MAX Set PIDF Constants.vi"("PID Constants"=w184, "MotorControlDeviceRef"=w183) -> ("MotorControlDeviceRef"=w185:T4)  [unwired: 8 in, 1 out]
          }
        }
        n70 = feedback-in #1(w172) -> ()
        n71 = Divide(x=w170, y=w168) -> (x/y=w169:dbl)
        n72 = call <vilib>:"Spark MAX Get Sensor Velocity.vi"("MotorControlDevRef in"=w180) -> ()  [unwired: 7 in, 4 out]
        n73 = call <vilib>:"Spark MAX Get Applied Output.vi"("MotorControlDevRef in"=w180) -> ()  [unwired: 7 in, 4 out]
        n74 = call <vilib>:"Spark MAX Set Output Advanced.vi"("Control Mode"=Spark_MAX_Control_Type."Position", "Setpoint"=w169, "MotorControlDevRef"=w180) -> ()  [unwired: 7 in, 2 out]
      }
    }
    n75 = case shown="\"on\"" w153 {
      tunnel: [w361 w364 -1.0 ("Output")] -> w152
      tunnel: w50 -> [_ w363 _]
      tunnel: w31 -> [w359 _ _]
      frame "on" {
        n76 = Select(t=0.9 ("Output"), s=w359, f=0.0) -> (s? t:f=w361:dbl)
      }
      frame "off", Default {
        n77 = Select(t=0.5 ("Output"), s=w363, f=0.0) -> (s? t:f=w364:dbl)
      }
      frame "reverse" {
      }
    }
    n78 = call <vilib>:"Spark MAX Get Sensor Position.vi"("MotorControlDevRef in"=w150) -> ("Sensor Position"=w145:dbl, "MotorControlDevRef out"=w139:T4)  [unwired: 7 in, 2 out]
    n79 = Negate(x="Inches per volt") -> (-x=w127:dbl)
    n80 = Multiply(x=w127, y=w39) -> (x*y=w131:dbl)
    n81 = Multiply(x=w127, y=w38) -> (x*y=w130:dbl)
    n82 = Multiply(x="clicks per inch arm", y=w145) -> (x*y=w136:dbl)
    n83 = case shown="\"protect\"" w157 {
      tunnel: ["Ground" "climb" "control panel" "protect"] -> w142
      frame "ground", Default {
      }
      frame "climb" {
      }
      frame "control panel" {
      }
      frame "protect" {
      }
    }
    n84 = call <vilib>:"WPI_MotorControlSetOutput.vi"("Output"=w152, "MotorControlDevRef"=w151) -> ()  [unwired: 7 in, 3 out]
    n85 = global read "GlobalVariables.vi" "Shooter Wheels"() -> (w140:enum16{"on", "off"})
    n86 = Negate(x=w136) -> (-x=w135:dbl)
    "Arm Extension Encoder" <- w135
    n87 = In Range and Coerce(upper limit=19.0, x=w61, lower limit=0.0) -> (coerced(x)=w60:dbl)  [unwired: 1 out]
    n88 = Multiply(x="Inches per volt", y="right act value at 1 inch") -> (x*y=w129:dbl)
    n89 = Add(x=w129, y=w130) -> (x+y=w44:dbl)
    "right act pos" <- w44
    n90 = case shown="\"on\"" w140 {
      tunnel: ["setpoint" 0.0 ("setpoint")] -> w85
      frame "on" {
      }
      frame "off", Default {
      }
    }
    n91 = local read "Crash Avoidance"() -> (w33:bool)
    n92 = global read "GlobalVariables.vi" "Turret Preset"() -> (w34:enum16{"free track", "forward", "backward"})
    n93 = Multiply(x="Inches per volt", y="left act value at 1 inch") -> (x*y=w132:dbl)
    n94 = global write "GlobalVariables.vi" "Hood Setpoint"(w88) -> ()
    n95 = Add(x=w132, y=w131) -> (x+y=w42:dbl)
    "left act pos" <- w42
    n96 = call-poly <vilib>:"PID.vi"("output range"=cluster{"output high":dbl, "output low":dbl} {"output high"=1.0, "output low"=-1.0}, "PID gains"="Arm Extension Gains", "process variable"=w135, "setpoint"=w60) -> ("output"=w148:dbl)  [unwired: 6 in, 1 out]
    n97 = global write "GlobalVariables.vi" "Linear Acuator Setpoint"(w142) -> ()
    n98 = Select(t=enum16{"free track", "forward", "backward"}."backward" ("f"), s=w33, f=w34) -> (s? t:f=w36:enum16{"free track", "forward", "backward"})
    n99 = Negate(x=w148) -> (-x=w137:dbl)
    n100 = In Range and Coerce(upper limit=w40, x=w38, lower limit=w43) -> (In Range?=w47:bool)  [unwired: 1 out]
    n101 = disable-structure shown="Enabled" {
      disable-tunnel: w118 -> [w241 _]
      disable-tunnel: w85 -> [w233 w245]
      disable-tunnel: w81 -> [w231 w248]
      frame Disabled {
        n102 = call <vilib>:"WPI_EncoderGet.vi"("EncoderDevRef"=w241) -> ("Rate"=w243:dbl)  [unwired: 5 in, 5 out]
        n103 = Divide(x=w243, y=6.0) -> (x/y=w238:dbl)
        "RPM" <- w238
        n104 = global write "GlobalVariables.vi" "RPM"(w238) -> ()
        n105 = Add(x=w233, y=50.0) -> (x+y=w236:dbl)
        n106 = Subtract(x=w233, y=50.0) -> (x-y=w234:dbl)
        n107 = In Range and Coerce(upper limit=w236, x=w238, lower limit=w234) -> (In Range?=w237:bool)  [unwired: 1 out]
        n108 = global write "GlobalVariables.vi" "Shooter in range?"(w237) -> ()
        n109 = call-poly <vilib>:"PID.vi"("output range"=cluster{"output high":dbl, "output low":dbl} {"output high"=0.9, "output low"=0.0}, "PID gains"="Shooter Gains", "process variable"=w238, "setpoint"=w233) -> ("output"=w230:dbl)  [unwired: 6 in, 1 out]
        n110 = call <vilib>:"WPI_MotorControlSetOutput.vi"("Output"=w230, "MotorControlDevRef"=w231) -> ()  [unwired: 7 in, 3 out]
      }
      frame Enabled {
        n111 = feedback #2(T1 {"P Gain"=0.0, "I Gain"=0.0, "D Gain"=0.0, "F Gain"=0.0, "I Zone"=0.0, "Min Output"=0.0, "Max Output"=0.0} ("PID Constants")) -> (w257:T1)
        n112 = Not Equal?(x="PID Constants shooter", y=w257) -> (x != y?=w253:T25)
        n113 = Cluster To Array(cluster=w253) -> (array=w254:bool[])
        n114 = Or Array Elements(Boolean array=w254) -> (logical OR=w255:bool)
        n115 = case shown="True" w255 {
          tunnel: "PID Constants shooter" -> [_ w261]
          tunnel: [w259 w261] -> w249
          tunnel: w257 -> [w259 _]
          tunnel: [w258 w262] -> w252
          tunnel: w248 -> [w258 w260]
          frame False {
          }
          frame True {
            n116 = call <vilib>:"Spark MAX Set PIDF Constants.vi"("PID Constants"=w261, "MotorControlDeviceRef"=w260) -> ("MotorControlDeviceRef"=w262:T4)  [unwired: 8 in, 1 out]
          }
        }
        n117 = feedback-in #2(w249) -> ()
        n118 = call <vilib>:"Spark MAX Get Sensor Velocity.vi"("MotorControlDevRef in"=w252) -> ("Sensor Velocity"=w246:dbl)  [unwired: 7 in, 3 out]
        "Sensor Velocity" <- w246
        n119 = call <vilib>:"Spark MAX Get Applied Output.vi"("MotorControlDevRef in"=w252) -> ()  [unwired: 7 in, 4 out]
        n120 = Greater Or Equal?(x=w246, y="min RPM") -> (x >= y?=w244:bool)
        "Shooter in range?" <- w244
        n121 = call <vilib>:"Spark MAX Set Output Advanced.vi"("Control Mode"=Spark_MAX_Control_Type."Velocity", "Setpoint"=w245, "MotorControlDevRef"=w252) -> ()  [unwired: 7 in, 2 out]
        n122 = global write "GlobalVariables.vi" "Shooter in range?"(w244) -> ()
      }
    }
    n123 = call <vilib>:"WPI_MotorControlSetOutput.vi"("Output"=w137, "MotorControlDevRef"=w139) -> ()  [unwired: 7 in, 3 out]
    n124 = In Range and Coerce(upper limit=w40, x=w39, lower limit=w43) -> (In Range?=w45:bool)  [unwired: 1 out]
    n125 = global write "GlobalVariables.vi" "Limelight Target Found?"(w32) -> ()
    n126 = Or(x=w45, y=w47) -> (x .or. y?=w46:bool)
    n127 = case shown="False" w46 {
      tunnel: w44 -> [_ w189]
      tunnel: [w187 w189] -> w48
      tunnel: w42 -> [_ w188]
      tunnel: [w186 w188] -> w41
      frame False {
        n128 = global read "GlobalVariables.vi" "Arm Height Pot Right"() -> (w187:dbl)
        n129 = global read "GlobalVariables.vi" "Arm Height Pot Left"() -> (w186:dbl)
      }
      frame True {
      }
    }
    n130 = global write "GlobalVariables.vi" "Arm Height Pot Left"(w41) -> ()
    n131 = global write "GlobalVariables.vi" "Arm Height Pot Right"(w48) -> ()
    n132 = call <vilib>:"Spark MAX Get Sensor Position.vi"("MotorControlDevRef in"=w138) -> ("Sensor Position"=w117:dbl, "MotorControlDevRef out"=w113:T4)  [unwired: 7 in, 2 out]
    n133 = global read "GlobalVariables.vi" "Linear Acuator Setpoint"() -> (w122:dbl)
    n134 = call-poly <vilib>:"PID.vi"("output range"=w119, "PID gains"="Acuator Gains", "process variable"=w41, "setpoint"=w122) -> ("output"=w121:dbl)  [unwired: 6 in, 1 out]
    n135 = call <vilib>:"WPI_MotorControlSetOutput.vi"("Output"=w121, "MotorControlDevRef"=w120) -> ()  [unwired: 7 in, 3 out]
    n136 = Multiply(x="degrees per click turret", y=w117) -> (x*y=w93:dbl)
    "turret degrees" <- w93
    n137 = case shown="\"free track\"" w36 {
      tunnel: ["Forward" "Backward" w322] -> w112
      tunnel: [0.0 ("Limelight LED State") 0.0 ("Limelight LED State") 0.0 ("Limelight LED State")] -> w110
      tunnel: [w310 "Backward" w325] -> w100
      tunnel: w93 -> [w309 w316 _]
      tunnel: [w309 w316 w323] -> w98
      tunnel: [1.0 ("Numeric") 1.0 ("Numeric") 0.0 ("Numeric")] -> w107
      tunnel: [0.0 ("Numeric") 0.0 ("Numeric") w321] -> w96
      tunnel: [1.0 ("Numeric") 1.0 ("Numeric") 3.0 ("Numeric")] -> w82
      tunnel: w32 -> [_ _ w319]
      frame "forward" {
        n138 = global read "GlobalVariables.vi" "Turret Setpoint"() -> (w310:dbl)
      }
      frame "backward", Default {
      }
      frame "free track" {
        # "tx = Horizontal Offset From Crosshair To Target (-27 degrees to 27 degrees)\nty = Vertical Offset From Crosshair To Target (-20.5 degrees to 20.5 degrees) \nta = Target Area (0% of image to 100% of image)\nts = Rotation or “skew” of your target \ntv = Whether the limelight has any valid targets (0 or 1)"
        n139 = call-poly <vilib>:"NT Read Value.vi"("Name"="/limelight/tx") -> ("Numeric"=w321:dbl)  [unwired: 9 in, 1 out]
        n140 = case shown="1" w319 {
          tunnel: [w329 0.0 ("Backward")] -> w325
          tunnel: [w329 w337] -> w323
          tunnel: [w328 w336] -> w322
          tunnel: w321 -> [_ w330]
          frame 0, Default {
            w329 = 0.0 ("Backward")
            n141 = global read "GlobalVariables.vi" "Turret Setpoint"() -> (w328:dbl)
          }
          frame 1 {
            n142 = Negate(x="X Accepted Range Turret") -> (-x=w333:dbl)
            n143 = In Range and Coerce(upper limit="X Accepted Range Turret", x=w330, lower limit=w333) -> (In Range?=w335:bool)  [unwired: 1 out]
            n144 = Multiply(x=w330, y="Auto Correct Gain Turret") -> (x*y=w337:dbl)
            n145 = Select(t="Minimum Track Value Turret", s=w335, f=w337) -> (s? t:f=w336:dbl)
          }
        }
      }
    }
    n146 = global write "GlobalVariables.vi" "Turret Encoder Value"(w93) -> ()
    n147 = call-poly <vilib>:"PID.vi"("output range"=w119, "PID gains"="Acuator Gains", "process variable"=w48, "setpoint"=w122) -> ("output"=w124:dbl)  [unwired: 6 in, 1 out]
    n148 = Less?(x=w96, y=w97) -> (x < y?=w95:bool)
    n149 = Greater Or Equal?(x=w93, y="upper limit") -> (x >= y?=w105:bool)
    n150 = Less Or Equal?(x=w93, y="lower limit") -> (x <= y?=w106:bool)
    n151 = Greater Or Equal?(x=w96, y=w97) -> (x >= y?=w94:bool)
    n152 = call <vilib>:"WPI_MotorControlSetOutput.vi"("Output"=w124, "MotorControlDevRef"=w125) -> ()  [unwired: 7 in, 3 out]
    n153 = Build Array(w94, w95, w106, w105) -> (w104:bool[])
    n154 = Boolean Array To Number(Boolean array=w104) -> (number=w103:u32)
    n155 = call <vilib>:"Color Sensor V3 Get Color.vi"("ColorSensorDevRef"=w84) -> ("error out"=w75:errorcluster, "Normalized Color"=w77:cluster{"R":dbl, "G":dbl, "B":dbl}, "Color"=→"Color":u32, "ColorSensorDevRef out"=w79:T15)  [unwired: 7 in]
    "Measured Color" <- w77
    n156 = global write "GlobalVariables.vi" "Turret Setpoint"(w112) -> ()
    n157 = case shown="6" w103 {
      tunnel: [w301 0.0 w303 w304 0.0] -> w99
      tunnel: w98 -> [w301 _ w303 w304 _]
      frame 0..3, Default {
      }
      frame 5 {
      }
      frame 6 {
      }
      frame 9 {
      }
      frame 10 {
      }
    }
    n158 = call-poly <vilib>:"NT Write Value.vi"("Numeric"=w110, "Name"="/limelight/pipeline") -> ()  [unwired: 9 in, 1 out]
    n159 = call <vilib>:"Color Sensor V3 Get Proximity.vi"("error in (no error)"=w75, "ColorSensorDevRef"=w79) -> ("Proximity"=→"Proximity":u16)  [unwired: 7 in, 2 out]
    n160 = call-poly <vilib>:"NT Write Value.vi"("Numeric"=w82, "Name"="/limelight/ledMode") -> ()  [unwired: 9 in, 1 out]
    n161 = call-poly <vilib>:"NT Write Value.vi"("Numeric"=w107, "Name"="/limelight/camMode") -> ()  [unwired: 9 in, 1 out]
    n162 = call <vilib>:"Color Sensor V3 Match Color.vi"("Measured Color"=w77) -> ("Confidence"=→"Confidence":dbl, "Matched Color Name"=w72:string)  [unwired: 8 in, 1 out]
    "Matched Color Name" <- w72
    n163 = global read "GlobalVariables.vi" "Intake State"() -> (w141:enum16{"Idle", "Intake", "Spit"})
    n164 = call-poly <vilib>:"PID.vi"("output range"=cluster{"output high":dbl, "output low":dbl} {"output high"=1.0, "output low"=-1.0}, "PID gains"="Turret Gains", "process variable"=w99, "setpoint"=w100) -> ("output"=w114:dbl)  [unwired: 6 in, 1 out]
    n165 = case shown="\"Idle\", Default" w141 {
      tunnel: [w351 -1.0 ("Output") 0.0 ("Output")] -> w68
      frame "Intake" {
        n166 = global read "GlobalVariables.vi" "Linear Acuator Setpoint"() -> (w344:dbl)
        n167 = global read "GlobalVariables.vi" "Linear Acuator Setpoint"() -> (w346:dbl)
        n168 = global read "GlobalVariables.vi" "Positional Achieved?"() -> (w349:bool)
        n169 = global read "GlobalVariables.vi" "Rotational Achieved?"() -> (w350:bool)
        n170 = Subtract(x=w346, y="control panel lin act offset") -> (x-y=w345:dbl)
        n171 = Or(x=w350, y=w349) -> (x .or. y?=w348:bool)
        n172 = case shown="False" w348 {
          tunnel: [0.5 ("t") 0.0 ("t")] -> w347
          frame False {
          }
          frame True {
          }
        }
        n173 = global read "GlobalVariables.vi" "Robot States"() -> (w354:T22)
        n174 = Equal?(x=w354, y=T22."control panel" ("Robot States")) -> (x = y?=w341:bool)
        n175 = Select(t=w345, s=w341, f=w344) -> (s? t:f=w343:dbl)
        n176 = global write "GlobalVariables.vi" "Linear Acuator Setpoint"(w343) -> ()
        n177 = Select(t=w347, s=w341, f=1.0) -> (s? t:f=w351:dbl)
      }
      frame "Spit" {
      }
      frame "Idle", Default {
      }
    }
    n178 = global read "GlobalVariables.vi" "Control Panel Mode"() -> (w73:enum16{"Rotational", "None", "Posistional"})
    n179 = global read "GlobalVariables.vi" "Rotation Counter"() -> (w74:dbl)
    n180 = call <vilib>:"WPI_MotorControlSetOutput.vi"("Output"=w114, "MotorControlDevRef"=w113) -> ()  [unwired: 7 in, 3 out]
    n181 = call <vilib>:"WPI_DriverStationGame Specific Data.vi"() -> ("Game Specific Data"=w69:string)  [unwired: 11 in]
    n182 = case shown="\"Rotational\", Default" w73 {
      tunnel: w74 -> [w200 _ _]
      tunnel: w72 -> [w202 w219 _]
      tunnel: w71 -> [w194 w214 _]
      tunnel: [w199 w214 FALSE ("x")] -> w70
      tunnel: w69 -> [_ w220 _]
      tunnel: [w192 w216 FALSE] -> w67
      tunnel: [w191 w215 0.0] -> w66
      tunnel: [w190 w217 FALSE ("Positional Achieved?")] -> w65
      frame "Rotational", Default {
        n183 = Equal?(x=FALSE, y=w194) -> (x = y?=w197:bool)
        n184 = Equal?(x="Yellow", y=w202) -> (x = y?=w195:bool)
        n185 = And(x=w195, y=w197) -> (x .and. y?=w196:bool)
        n186 = case shown="False" w196 {
          tunnel: w200 -> [w210 w213]
          tunnel: [w208 w212] -> w191
          tunnel: [w206 TRUE] -> w199
          tunnel: w195 -> [w207 _]
          tunnel: w194 -> [w204 _]
          frame False {
            n187 = Not(x=w207) -> (.not. x?=w205:bool)
            n188 = Add(x=w210, y=0.0) -> (x+y=w208:dbl)
            n189 = Select(t=FALSE, s=w205, f=w204) -> (s? t:f=w206:bool)
          }
          frame True {
            n190 = Increment(x=w213) -> (x+1=w212:dbl)
          }
        }
        n191 = global read "GlobalVariables.vi" "Positional Achieved?"() -> (w190:bool)
        n192 = Greater Or Equal?(x=7.0, y=w191) -> (x >= y?=w192:bool)
      }
      frame "Posistional" {
        n193 = case shown="\"empty\", Default" w220 {
          tunnel: ["empty" "Red" "Green" "Blue" "Yellow"] -> w218
          frame "empty", Default {
          }
          frame "R" {
          }
          frame "G" {
          }
          frame "B" {
          }
          frame "Y" {
          }
        }
        n194 = Equal?(x=w218, y=w219) -> (x = y?=w217:bool)
        n195 = global read "GlobalVariables.vi" "Rotational Achieved?"() -> (w216:bool)
        n196 = global read "GlobalVariables.vi" "Rotation Counter"() -> (w215:dbl)
      }
      frame "None" {
      }
    }
    n197 = call <vilib>:"WPI_MotorControlSetOutput.vi"("Output"=w68, "MotorControlDevRef"=w144) -> ()  [unwired: 7 in, 3 out]
    n198 = global write "GlobalVariables.vi" "Rotation Counter"(w66) -> ()
    n199 = global write "GlobalVariables.vi" "Positional Achieved?"(w65) -> ()
    n200 = global write "GlobalVariables.vi" "Rotational Achieved?"(w67) -> ()
  }
  n201 = while {
    stop <- FALSE stop-if-true
    # "100 ms tasks go here"
    n202 = Wait (ms)(milliseconds to wait=u32 100) -> ()  [unwired: 1 out]
    n203 = global read "GlobalVariables.vi" "Robot States"() -> (w390:T22)
    n204 = case shown="\"unjam\"" w390 {
      tunnel: [T24."protect" ("Arm Height") T24."ground" ("Arm Height") w414 T24."protect" ("Arm Height") w436 T24."ground" ("Arm Height") T24."ground" ("Arm Height")] -> w389
      tunnel: [T23."protect" ("Arm Extension") T23."intake" ("Arm Extension") w413 T23."protect" ("Arm Extension") w435 T23."intake" ("Arm Extension") T23."intake" ("Arm Extension")] -> w388
      tunnel: [w393 w401 w409 w423 w431 w445 w453] -> w387
      frame "ground protect", Default {
        n205 = global read "GlobalVariables.vi" "Arm Height Pot Right"() -> (w397:dbl)
        n206 = Less Or Equal?(x=w397, y=0.3) -> (x <= y?=w398:bool)
        n207 = case shown="True" w398 {
          tunnel: [TRUE ("Crash Avoidance") FALSE ("Crash Avoidance")] -> w393
          frame False {
          }
          frame True {
          }
        }
      }
      frame "ground pickup" {
        n208 = global read "GlobalVariables.vi" "Arm Height Pot Right"() -> (w405:dbl)
        n209 = Less Or Equal?(x=w405, y=0.3) -> (x <= y?=w406:bool)
        n210 = case shown="False" w406 {
          tunnel: [TRUE ("Crash Avoidance") FALSE ("Crash Avoidance")] -> w401
          frame False {
          }
          frame True {
          }
        }
      }
      frame "control panel" {
        n211 = global read "GlobalVariables.vi" "Turret Encoder Value"() -> (w416:dbl)
        n212 = local read "upper limit"() -> (w412:dbl)
        n213 = Subtract(x=w412, y=5.0) -> (x-y=w410:dbl)
        n214 = Greater Or Equal?(x=w416, y=w410) -> (x >= y?=w415:bool)
        n215 = case shown="True" w415 {
          tunnel: [w419 T24."control panel" ("Arm Height")] -> w414
          tunnel: [T23."intake" ("Arm Extension") T23."control" ("Arm Extension")] -> w413
          tunnel: [TRUE ("Crash Avoidance") TRUE ("Crash Avoidance")] -> w409
          frame False {
            (unwired) enum16{"free track", "forward", "backward"}."backward" ("Turret Preset")
            n216 = global read "GlobalVariables.vi" "Arm Height"() -> (w419:T24)
          }
          frame True {
          }
        }
      }
      frame "shooting" {
        n217 = global read "GlobalVariables.vi" "Arm Height Pot Right"() -> (w428:dbl)
        n218 = Less Or Equal?(x=w428, y=0.3) -> (x <= y?=w426:bool)
        n219 = case shown="False" w426 {
          tunnel: [TRUE ("Crash Avoidance") FALSE ("Crash Avoidance")] -> w423
          frame False {
          }
          frame True {
          }
        }
      }
      frame "climb" {
        n220 = global read "GlobalVariables.vi" "Turret Encoder Value"() -> (w438:dbl)
        n221 = local read "upper limit"() -> (w434:dbl)
        n222 = Subtract(x=w434, y=5.0) -> (x-y=w432:dbl)
        n223 = Greater Or Equal?(x=w438, y=w432) -> (x >= y?=w437:bool)
        n224 = case shown="True" w437 {
          tunnel: [w441 T24."climb" ("Arm Height")] -> w436
          tunnel: [w440 T23."climb" ("Arm Extension")] -> w435
          tunnel: [TRUE TRUE] -> w431
          frame False {
            n225 = global read "GlobalVariables.vi" "Arm Extension"() -> (w440:T23)
            n226 = global read "GlobalVariables.vi" "Arm Height"() -> (w441:T24)
          }
          frame True {
          }
        }
      }
      frame "unjam" {
        n227 = global read "GlobalVariables.vi" "Arm Height Pot Right"() -> (w450:dbl)
        n228 = Less Or Equal?(x=w450, y=0.3) -> (x <= y?=w448:bool)
        n229 = case shown="False" w448 {
          tunnel: [TRUE ("Crash Avoidance") FALSE ("Crash Avoidance")] -> w445
          frame False {
          }
          frame True {
          }
        }
      }
      frame "intake shoot" {
        n230 = global read "GlobalVariables.vi" "Arm Height Pot Right"() -> (w457:dbl)
        n231 = Less Or Equal?(x=w457, y=0.3) -> (x <= y?=w458:bool)
        n232 = case shown="True" w458 {
          tunnel: [TRUE ("Crash Avoidance") FALSE ("Crash Avoidance")] -> w453
          frame False {
          }
          frame True {
          }
        }
      }
    }
    "Crash Avoidance" <- w387
    n233 = global write "GlobalVariables.vi" "Arm Extension"(w388) -> ()
    n234 = global write "GlobalVariables.vi" "Arm Height"(w389) -> ()
  }
